vi "lauda_test.vi"() -> ()   [LabVIEW 2015]
uses:
  BERTTA.dll
panel:
  in  "set_temp":dbl
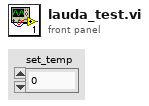
[diagram p1: front panel]
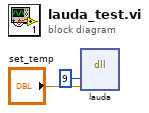
[diagram p0: block diagram]
diagram:
  n1 = dll-call lib="C:/Users/shresplab/OneDrive - Kemira Oyj/Documents/Visual Studio 2017/Projects/Bertta/BERTTA/x64/Debug/BERTTA.dll" fn="lauda"("port"=9, "set_temp"="set_temp") -> ()  [unwired: 6 in, 2 out]
